vi "ExecuteRole.vi"(0 "object in":refnum<class "SupportAttackerRole.lvclass">, 2 "Robot in":refnum<class "Robot.lvclass">, 3 "GameRef":refnum<data-value>, 5 "error in (no error)":errorcluster) -> (14 "object out":refnum<class "SupportAttackerRole.lvclass">, 16 "Robot out":refnum<class "Robot.lvclass">, 19 "error out":errorcluster)   [LabVIEW 2023, in "SupportAttackerRole.lvclass"]
uses:
  SupportAttackerRole.lvclass
  C:/Users/ebert/Documents/codes/SSL/repo/SSL_AI/NewSTP/NewRoles/Role_v2_class/Role_v2.lvclass
  Robot_class/Robot.lvclass
  Game_class/Game.lvclass
  SupportAttackerRole_states.ctl
  NewSTP/NewRoles/Role_v2_class/Role_v2.lvclass
  Zone_class/Zone.lvclass
  NewSTP/Evaluators/Evaluator_class/Evaluator.lvclass
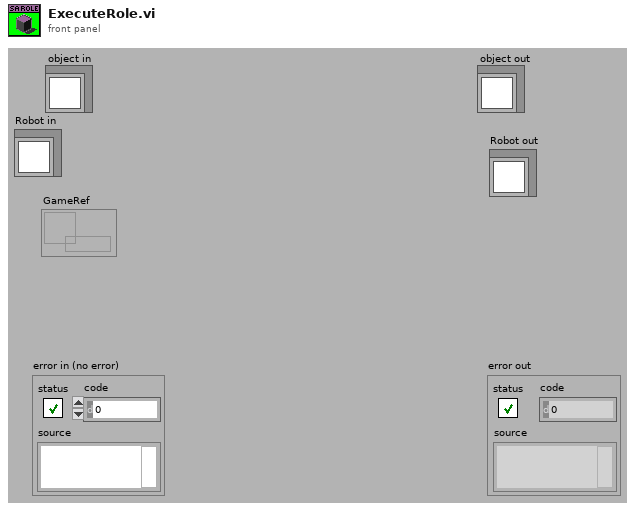
[diagram p1: front panel]
types:
  T1 = typedef "SupportAttackerRole.lvclass/SupportAttackerRole_states.ctl" = enum16{"Position", "WaitPass", "Exit"}
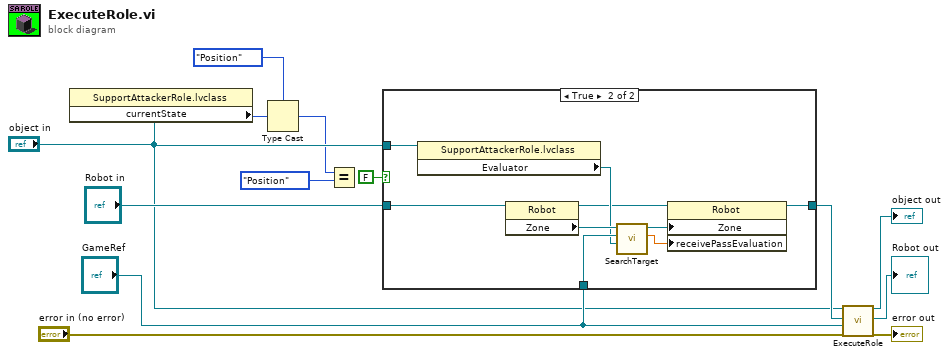
[diagram p0: block diagram]
diagram:
  n1 = property class="SupportAttackerRole.lvclass"(reference="object in") -> ("currentState"=w5:u8)  [unwired: 1 in, 2 out]
  n2 = Type Cast(type=SupportAttackerRole_states."Position" ("States"), x=w5) -> (*(type *) &x=w4:T1)
  n3 = Equal?(x=w4, y=SupportAttackerRole_states."Position" ("States")) -> ()  [unwired: 1 out]
  n4 = case shown="True" FALSE {
    tunnel: "object in" -> [_ w23]
    tunnel: "Robot in" -> [w14 w22]
    tunnel: "GameRef" -> [_ w20]
    tunnel: [w14 w15] -> w7
    frame False {
    }
    frame True {
      n5 = property class="SupportAttackerRole.lvclass"(reference=w23) -> ("Evaluator"=w19:refnum<class "Evaluator.lvclass">)  [unwired: 1 in, 2 out]
      n6 = property class="Robot"(reference=w22) -> (reference out=w18:refnum<class "Robot.lvclass">, "Zone"=w21:refnum<class "Zone.lvclass">)  [unwired: 1 in, 1 out]
      n7 = call-dynamic "SearchTarget.vi"("Evaluator"=w19, "GameRef"=w20, "object in"=w21) -> ("receiverEval"=w16:dbl, "object out"=w17:refnum<class "Zone.lvclass">)  [unwired: 6 in, 1 out]
      n8 = property class="Robot"(reference=w18, "Zone"=w17, "receivePassEvaluation"=w16) -> (reference out=w15:refnum<class "Robot.lvclass">)  [unwired: 1 in, 1 out]
    }
  }
  n9 = call-parent "ExecuteRole.vi"("object in"="object in", "Robot in"=w7, "GameRef"="GameRef", "error in (no error)"="error in (no error)") -> ("object out"=→"object out":refnum<class "SupportAttackerRole.lvclass">, "Robot out"=→"Robot out":refnum<class "Robot.lvclass">, "error out"=→"error out":errorcluster)  [unwired: 13 in]
